vi "AMC Check Message Queue Status.vi"(7 "error in (no error)":errorcluster, 10 "Message queue in":T1) -> (0 "error out":errorcluster, 2 "# elements in queue":i32, 3 "Message queue out":T1)   [LabVIEW 2009]
doc: "This VI is used for compatibility with previous versions of the AMC library. Use the AMC VIs located in the <b>Data Communication >> Asynchronous Message Communication</b> palette."
uses:
  Message Queue.ctl
  Message.ctl
  <vilib>/NI/Tools/Keyed Array/KeyedArray.ctl
  AMC.lvlib
  <vilib>/NI/Tools/Keyed Array/Tools_KeyedArray.lvlib
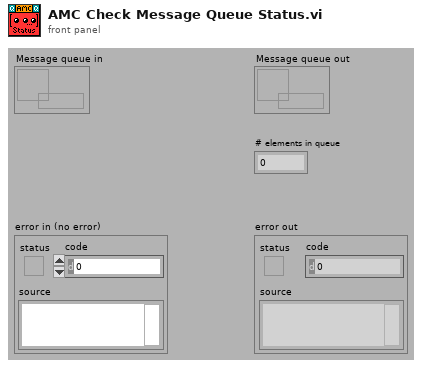
[diagram p1: front panel]
types:
  T1 = typedef "AMC.lvlib/Message Queue.ctl" = refnum<queue>
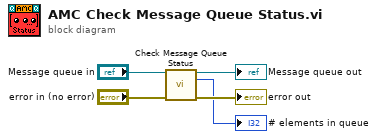
[diagram p0: block diagram]
diagram:
  n1 = call "Check Message Queue Status.vi"("message queue in"="Message queue in", "error in"="error in (no error)") -> ("message queue out"=→"Message queue out":T1, "# elements in queue"=→"# elements in queue":i32, "error out"=→"error out":errorcluster)  [unwired: 9 in, 2 out]
